vi "PCU_Connect.vi"(1 "Address/ComPort":string, 2 "Communication":T1(ring), 3 "Terminator":enum32{"Cr", "Lf", "CrLf"}(ring), 4 "Portnumber":i32, 5 "error in":errorcluster) -> (14 "Reference out":refnum<k24>, 19 "error out":errorcluster)   [LabVIEW 2017]
uses:
  LV_IL_Sample/DLL/InstrumentDLL.dll
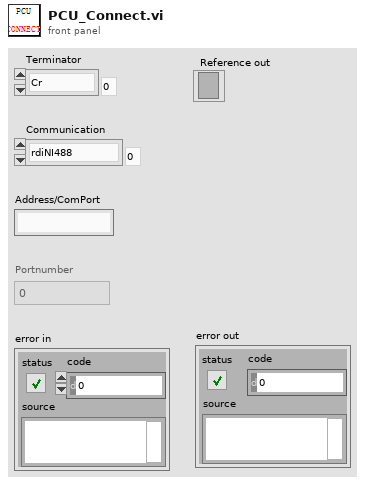
[diagram p1: front panel]
types:
  T1 = enum32{"rdiNI488", "rdiNIvisa", "rdikeysightvisa", "rdiUSB", "rdiLAN"}
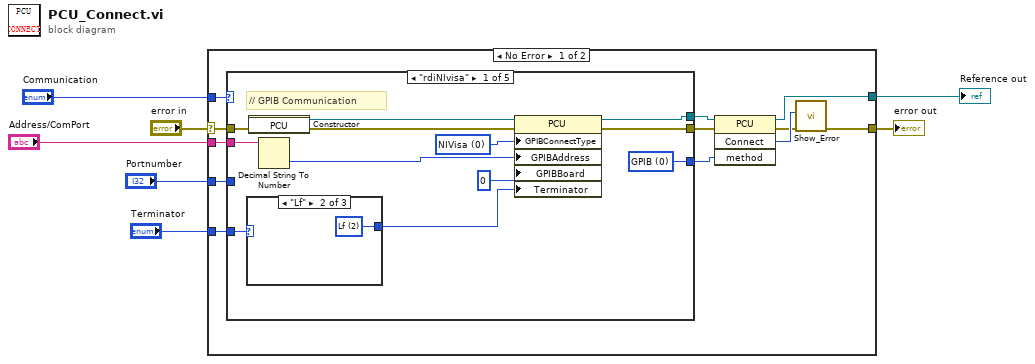
[diagram p0: block diagram]
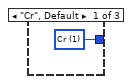
[diagram p2: hidden frame]
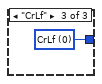
[diagram p3: hidden frame]
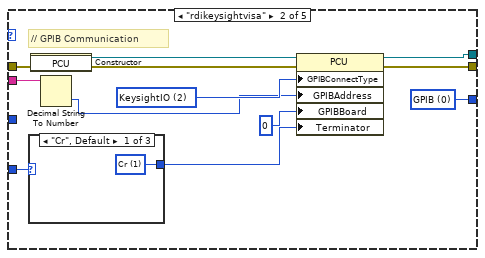
[diagram p4: hidden frame]
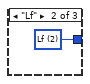
[diagram p5: hidden frame]
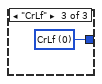
[diagram p6: hidden frame]
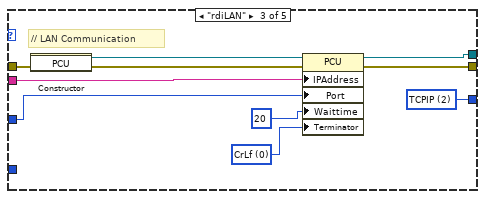
[diagram p7: hidden frame]
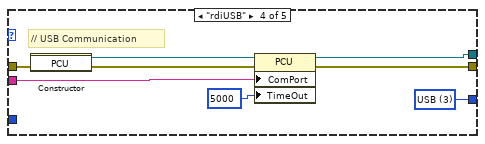
[diagram p8: hidden frame]
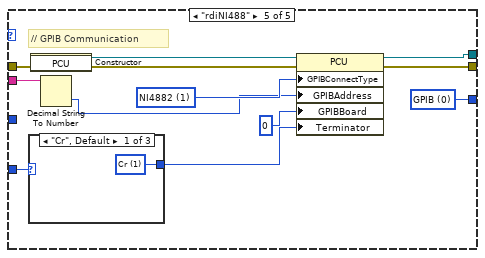
[diagram p9: hidden frame]
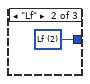
[diagram p10: hidden frame]
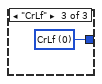
[diagram p11: hidden frame]
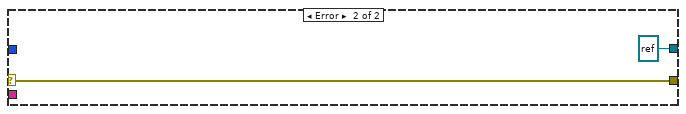
[diagram p12: hidden frame]
diagram:
  n1 = case shown="No Error" "error in" {
    selector: "error in" -> [w16 w84]
    tunnel: "Address/ComPort" -> [w19 _]
    tunnel: [w9 refnum<k24> refnum ("new reference")] -> w6
    tunnel: [w10 w84] -> w5
    tunnel: "Terminator" -> [w18 _]
    tunnel: "Communication" -> [w17 _]
    tunnel: "Portnumber" -> [w8 _]
    frame No Error {
      n2 = case shown="\"rdiNIvisa\"" w17 {
        tunnel: w19 -> [w29 w44 w59 w65 w77]
        tunnel: w16 -> [w26 w40 w57 w63 w73]
        tunnel: w18 -> [w21 w36 _ _ w69]
        tunnel: [w22 w39 w52 w60 w70] -> w15
        tunnel: [w23 w38 w53 w61 w71] -> w14
        tunnel: [w24 w37 w54 w62 w72] -> w13
        tunnel: w8 -> [_ _ w50 _ _]
        frame "rdiNIvisa" {
          w24 = 0 items=["GPIB", "C232C", "TCPIP", "USB"] ("method")
          w31 = 0 items=["NIVisa", "NI4882", "KeysightIO"] ("GPIBConnectType")
          # "// GPIB Communication"
          n3 = case shown="\"Lf\"" w21 {
            tunnel: [w32 w33 w34] -> w20
            frame "Cr", Default {
              w32 = 1 items=["CrLf", "Cr", "Lf"] ("Terminator")
            }
            frame "Lf" {
              w33 = 2 items=["CrLf", "Cr", "Lf"] ("Terminator")
            }
            frame "CrLf" {
              w34 = 0 items=["CrLf", "Cr", "Lf"] ("Terminator")
            }
          }
          n4 = constructor class="PCU"(error in=w26) -> (reference out=w28:refnum<k24>, error out=w25:errorcluster)  [unwired: 2 in, 1 out]
          n5 = Decimal String To Number(string=w29) -> (number=w30:i32)  [unwired: 2 in, 1 out]
          n6 = property on="属性节点" class="PCU"(reference=w28, error in=w25, "GPIBConnectType"=w31, "GPIBAddress"=w30, "GPIBBoard"=0, "Terminator"=w20) -> (reference out=w22:refnum<k24>, error out=w23:errorcluster)
        }
        frame "rdikeysightvisa" {
          w37 = 0 items=["GPIB", "C232C", "TCPIP", "USB"] ("method")
          w46 = 2 items=["NIVisa", "NI4882", "KeysightIO"] ("GPIBConnectType")
          # "// GPIB Communication"
          n7 = case shown="\"Cr\", Default" w36 {
            tunnel: [w47 w48 w49] -> w35
            frame "Cr", Default {
              w47 = 1 items=["CrLf", "Cr", "Lf"] ("Terminator")
            }
            frame "Lf" {
              w48 = 2 items=["CrLf", "Cr", "Lf"] ("Terminator")
            }
            frame "CrLf" {
              w49 = 0 items=["CrLf", "Cr", "Lf"] ("Terminator")
            }
          }
          n8 = constructor class="PCU"(error in=w40) -> (reference out=w43:refnum<k24>, error out=w41:errorcluster)  [unwired: 2 in, 1 out]
          n9 = Decimal String To Number(string=w44) -> (number=w45:i32)  [unwired: 2 in, 1 out]
          n10 = property on="属性节点" class="PCU"(reference=w43, error in=w41, "GPIBConnectType"=w46, "GPIBAddress"=w45, "GPIBBoard"=0, "Terminator"=w35) -> (reference out=w39:refnum<k24>, error out=w38:errorcluster)
        }
        frame "rdiLAN" {
          w51 = 0 items=["CrLf", "Cr", "Lf"] ("Terminator")
          w54 = 2 items=["GPIB", "C232C", "TCPIP", "USB"] ("method")
          # "// LAN Communication"
          n11 = constructor class="PCU"(error in=w57) -> (reference out=w58:refnum<k24>, error out=w56:errorcluster)  [unwired: 2 in, 1 out]
          n12 = property on="属性节点" class="PCU"(reference=w58, error in=w56, "IPAddress"=w59, "Port"=w50, "Waittime"=20, "Terminator"=w51) -> (reference out=w52:refnum<k24>, error out=w53:errorcluster)
        }
        frame "rdiUSB" {
          w62 = 3 items=["GPIB", "C232C", "TCPIP", "USB"] ("method")
          # "// USB Communication"
          n13 = constructor class="PCU"(error in=w63) -> (reference out=w67:refnum<k24>, error out=w64:errorcluster)  [unwired: 2 in, 1 out]
          n14 = property on="属性节点" class="PCU"(reference=w67, error in=w64, "ComPort"=w65, "TimeOut"=5000 ("BaudRate")) -> (reference out=w60:refnum<k24>, error out=w61:errorcluster)
        }
        frame "rdiNI488" {
          w72 = 0 items=["GPIB", "C232C", "TCPIP", "USB"] ("method")
          w79 = 1 items=["NIVisa", "NI4882", "KeysightIO"] ("GPIBConnectType")
          # "// GPIB Communication"
          n15 = case shown="\"Cr\", Default" w69 {
            tunnel: [w80 w81 w82] -> w68
            frame "Cr", Default {
              w80 = 1 items=["CrLf", "Cr", "Lf"] ("Terminator")
            }
            frame "Lf" {
              w81 = 2 items=["CrLf", "Cr", "Lf"] ("Terminator")
            }
            frame "CrLf" {
              w82 = 0 items=["CrLf", "Cr", "Lf"] ("Terminator")
            }
          }
          n16 = constructor class="PCU"(error in=w73) -> (reference out=w76:refnum<k24>, error out=w74:errorcluster)  [unwired: 2 in, 1 out]
          n17 = Decimal String To Number(string=w77) -> (number=w78:i32)  [unwired: 2 in, 1 out]
          n18 = property on="属性节点" class="PCU"(reference=w76, error in=w74, "GPIBConnectType"=w79, "GPIBAddress"=w78, "GPIBBoard"=0, "Terminator"=w68) -> (reference out=w70:refnum<k24>, error out=w71:errorcluster)
        }
      }
      n19 = invoke on="调用节点" class="PCU" method="Connect"(reference=w15, error in=w14, "method"=w13) -> (reference out=w9:refnum<k24>, error out=w11:errorcluster, "Connect"=w12:i32)  [unwired: 1 in, 1 out]
      n20 = call "Show_Error.vi"("error in (no error)"=w11, "Error"=w12) -> ("error out"=w10:errorcluster)  [unwired: 9 in]
    }
    frame Error {
    }
  }
  "Reference out" <- w6
  "error out" <- w5
